vi "Protection_2.vi"() -> ()   [LabVIEW 2016]
uses:
  <vilib>/rvi/interface/nirviOpenFPGA/nirviOpenFPGA.xnode
  <vilib>/rvi/interface/nirviReadWriteControl/nirviReadWriteControl.xnode
  <vilib>/addons/Electrical Power/Basic/NI_EP_Basic.lvlib
  <vilib>/addons/Electrical Power/Basic/Measurement/RMS (N Channels).vi
  <vilib>/rvi/interface/nirviCloseFPGA/nirviCloseFPGA.xnode
  <vilib>/addons/Electrical Power/Basic/Measurement/Fundamental Vector (N Channels).vi
  FPGA Bitfiles/IntelliRupter2_FPGATarget.lvbitx
  <vilib>/FPGAPlugInAG/cRIO-9039 (Sync)/niLvFpga_Open_cRIO-9039 (Sync).vi
  <vilib>/rvi/interface/common/dynamic/niFpgaDynamicAddResources.vi
  <vilib>/rvi/interface/Simulation/niFpgaSimulationCallBeginRW.vi
  <vilib>/rvi/errors/niLvFpgaAdjustHostInterfaceError.vi
  <vilib>/FPGAPlugInAG/Dynamic/niLvFpga_Close_Dynamic.vi
  <vilib>/addons/Electrical Power/Protection/Definite Time Delay/subVIs/fpga_Time Delay Cfg.ctl
  <vilib>/addons/Electrical Power/Protection/NI_EP_Protection_FPGA.lvlib
panel:
  out "sum 2":dbl
  out "sum":dbl
  out "y":dbl[](array[numeric])
  out "x":dbl[](array[numeric])
  out "current fundamental vectors":cdb[](array[numeric])
  out "voltage fundamental vectors":cdb[](array[numeric])
  out "I array":waveform(sgl)[](array[waveform])=[{"t0"=timestamp(3615968248.53045 s since 1904-01-01), "dt"=1.736111111111111e-05, "Y"=array[1000 elements]}, {"t0"=timestamp(3615968248.53045 s since 1904-01-01), "dt"=1.736111111111111e-05, "Y"=array[1000 elements]}, {"t0"=timestamp(3615968248.53045 s since 1904-01-01), "dt"=1.736111111111111e-05, "Y"=array[1000 elements]}]
  out "VL array":waveform(sgl)[](array[waveform])=[{"t0"=timestamp(3615968248.53045 s since 1904-01-01), "dt"=1.736111111111111e-05, "Y"=array[1000 elements], "attributes"=variant("channel"=variant(enum16{"Va L", "Vb L", "Vc L", "Ia", "Ib", "Ic", "Va R", "Vb R", "Vc R"} enum."Va L"))}, {"t0"=timestamp(3615968248.53045 s since 1904-01-01), "dt"=1.736111111111111e-05, "Y"=array[1000 elements], "attributes"=variant("channel"=variant(enum16{"Va L", "Vb L", "Vc L", "Ia", "Ib", "Ic", "Va R", "Vb R", "Vc R"} enum."Vb L"))}, {"t0"=timestamp(3615968248.53045 s since 1904-01-01), "dt"=1.736111111111111e-05, "Y"=array[1000 elements], "attributes"=variant("channel"=variant(enum16{"Va L", "Vb L", "Vc L", "Ia", "Ib", "Ic", "Va R", "Vb R", "Vc R"} enum."Vc L"))}]
  in  "RMS minimum\nvalues":T1={"VRMS values"=[0.5, 0.5, 0.5], "IRMS values"=[0.1, 0.09999999999999998, 0.09999999999999998]}
  in  "Manual trip":bool
  in  "Relay7":bool
  in  "Reclose?":bool
  in  "Recloser Settings":T2={"Magnitude Minimum"=0.1, "Magnitude difference level"=0.1, "Frequency difference level"=0.1, "Phase difference level"=5.0}
  in  "time delay settings":T3={"operate time [ms]"=10, "reset time [ms]"=10, "operate time compensation [ms]"=10}
  out "VR error":i32
  out "VL error":i32
  in  "UV Reset level":dbl
  in  "Undervoltage \npick-up level":dbl=-1.0
  in  "OC Reset level":dbl=2.0
  in  "Overcurrent\npick-up level":dbl=100.0
  out "I error":i32
  in  "stop":bool
  out "half cycle (samples)":i32=96
  out "basic calc interval":u16=57600
  # "Overcurrent reset level should\nbe lower than pick-up level\n\nUndervoltage reset level should \nbe higher than pick-up level"
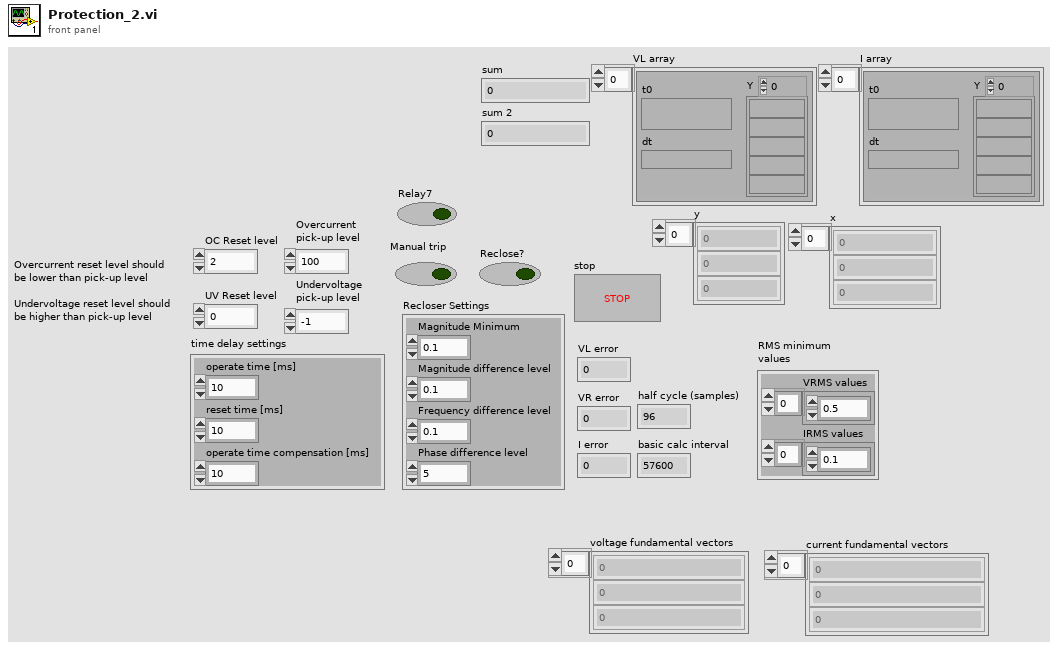
[diagram p1: front panel]
types:
  T1 = cluster{"VRMS values":dbl[], "IRMS values":dbl[]}
  T2 = cluster{"Magnitude Minimum":dbl, "Magnitude difference level":dbl, "Frequency difference level":dbl, "Phase difference level":dbl}
  T3 = typedef "NI_EP_Protection_FPGA.lvlib/fpga_Time Delay Cfg.ctl" = cluster{"operate time [ms]":u32, "reset time [ms]":u32, "operate time compensation [ms]":u32}
  T4 = typedef "NI_EP_Protection_FPGA.lvlib/fpga_Timer Feedback Var.ctl" = cluster{"time elapsed":u32, "start time of trip counting":u32, "start time of reseting":u32}
  T5 = typedef "NI_EP_Protection_FPGA.lvlib/fpga_State.ctl" = enum16{"Idle", "Trip Counting", "Tripped", "Reset Counting"}
  T6 = cluster{"timing values out":T4, "status out":T5, "trip signal out":bool}
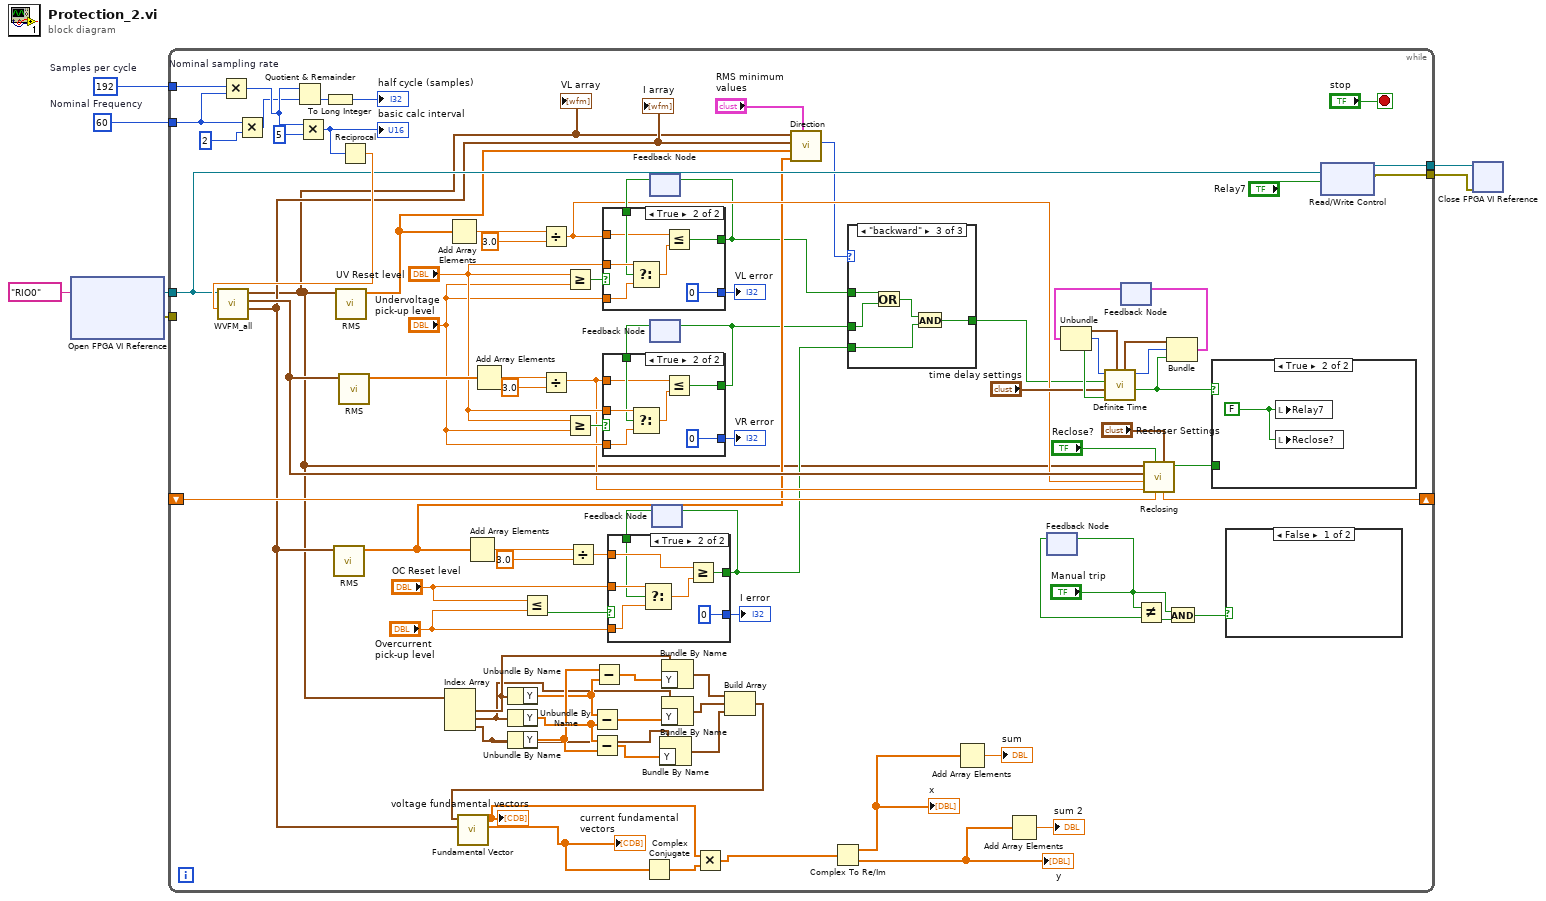
[diagram p0: block diagram]
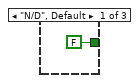
[diagram p2: hidden frame]
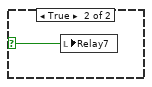
[diagram p5: hidden frame]
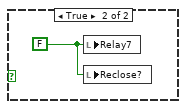
[diagram p6: hidden frame]
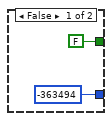
[diagram p7: hidden frame]
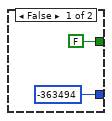
[diagram p8: hidden frame]
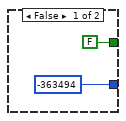
[diagram p9: hidden frame]
diagram:
  w3 = 192  # Samples per cycle
  w4 = 60  # Nominal Frequency
  n1 = xnode "Open FPGA VI Reference"("resource name"=tag "RIO0") -> ("FPGA VI Reference Out"=w7:refnum<k20>, "error out"=w6:errorcluster)  [unwired: 1 in]
  n2 = while {
    tunnel: w7 -> [w57]
    tunnel: w6 -> [_]
    tunnel: w4 -> [w88]
    tunnel: w3 -> [w87]
    shift-right: [w51] -> _
    shift-left: _ -> [w50]
    tunnel: [w49] -> w2
    tunnel: [w48] -> w1
    stop <- "stop" stop-if-true
    n3 = Multiply "Nominal sampling rate"(x=w87, y=w88) -> (x*y=w94:i32)
    n4 = Multiply(x=w88, y=2) -> (x*y=w90:i32)
    n5 = Quotient & Remainder(x=w94, y=w90) -> (floor(x/y)=w92:i32)  [unwired: 1 out]
    n6 = Multiply(x=w94, y=u16 5) -> (x*y=w95:i32)
    "basic calc interval" <- w95
    n7 = To Long Integer(number=w92) -> (32bit integer=→"half cycle (samples)":i32)
    n8 = Reciprocal(x=w95) -> (1/x=w85:dbl)
    n9 = call "WVFM_all.vi"("dt"=w85, "FPGA VI Reference"=w57) -> ("I array"=w30:waveform(sgl)[], "VR array"=w56:waveform(sgl)[], "VL array"=w15:waveform(sgl)[])  [unwired: 6 in]
    "VL array" <- w15
    "I array" <- w30
    n10 = call-poly <vilib>:"RMS.vi"("waveforms"=w30) -> ("RMS values"=w38:dbl[])  [unwired: 9 in, 1 out]
    n11 = call-poly <vilib>:"RMS.vi"("waveforms"=w15) -> ("RMS values"=w39:dbl[])  [unwired: 9 in, 1 out]
    n12 = call-poly <vilib>:"RMS.vi"("waveforms"=w56) -> ("RMS values"=w68:dbl[])  [unwired: 9 in, 1 out]
    n13 = Index Array(array=w15) -> (element #1=w23:waveform(sgl), element #2=w22:waveform(sgl), element #3=w20:waveform(sgl))  [unwired: 3 in]
    n14 = Add Array Elements(numeric array=w39) -> (sum=w76:dbl)
    n15 = Add Array Elements(numeric array=w38) -> (sum=w82:dbl)
    n16 = Add Array Elements(numeric array=w68) -> (sum=w71:dbl)
    n17 = Unbundle By Name(w23) -> ("Y"=w25:sgl[])
    n18 = Unbundle By Name(w22) -> ("Y"=w27:sgl[])
    n19 = Unbundle By Name(w20) -> ("Y"=w26:sgl[])
    n20 = Less Or Equal?(x="OC Reset level", y="Overcurrent\npick-up level") -> (x <= y?=w84:bool)
    n21 = Divide(x=w76, y=3.0) -> (x/y=w55:dbl)
    n22 = Divide(x=w71, y=3.0) -> (x/y=w54:dbl)
    n23 = Greater Or Equal?(x="UV Reset level", y="Undervoltage \npick-up level") -> (x >= y?=w79:bool)
    n24 = Greater Or Equal?(x="UV Reset level", y="Undervoltage \npick-up level") -> (x >= y?=w69:bool)
    n25 = Divide(x=w82, y=3.0 ("x")) -> (x/y=w81:dbl)
    n26 = Subtract(x=w25, y=w27) -> (x-y=w21:sgl[])
    n27 = Subtract(x=w27, y=w26) -> (x-y=w19:sgl[])
    n28 = Subtract(x=w26, y=w25) -> (x-y=w24:sgl[])
    n29 = feedback #1() -> (w77:bool)  [unwired: 1 in]
    n30 = case shown="True" w79 {
      tunnel: [FALSE w123] -> w35
      tunnel: [-363494 ("error") 0 ("error")] -> w74
      tunnel: "UV Reset level" -> [_ w121]
      tunnel: "Undervoltage \npick-up level" -> [_ w120]
      tunnel: w77 -> [_ w119]
      tunnel: w55 -> [_ w118]
      frame False {
      }
      frame True {
        n31 = Select(t=w121, s=w119, f=w120) -> (s? t:f=w124:dbl)
        n32 = Less Or Equal?(x=w118, y=w124) -> (x <= y?=w123:bool)
      }
    }
    "VL error" <- w74
    n33 = feedback-in #1(w35) -> ()
    n34 = feedback #2() -> (w70:bool)  [unwired: 1 in]
    n35 = case shown="True" w69 {
      tunnel: [FALSE w114] -> w34
      tunnel: [-363494 ("error") 0 ("error")] -> w73
      tunnel: "UV Reset level" -> [_ w112]
      tunnel: "Undervoltage \npick-up level" -> [_ w111]
      tunnel: w70 -> [_ w110]
      tunnel: w54 -> [_ w109]
      frame False {
      }
      frame True {
        n36 = Select(t=w112, s=w110, f=w111) -> (s? t:f=w115:dbl)
        n37 = Less Or Equal?(x=w109, y=w115) -> (x <= y?=w114:bool)
      }
    }
    "VR error" <- w73
    n38 = feedback-in #2(w34) -> ()
    n39 = feedback #3() -> (w78:bool)  [unwired: 1 in]
    n40 = case shown="True" w84 {
      tunnel: w81 -> [_ w133]
      tunnel: [-363494 ("error") 0 ("error")] -> w83
      tunnel: "OC Reset level" -> [_ w130]
      tunnel: "Overcurrent\npick-up level" -> [_ w129]
      tunnel: [FALSE ("Boolean") w128] -> w33
      tunnel: w78 -> [_ w127]
      frame False {
      }
      frame True {
        n41 = Select(t=w130, s=w127, f=w129) -> (s? t:f=w132:dbl)
        n42 = Greater Or Equal?(x=w133, y=w132) -> (x >= y?=w128:bool)
      }
    }
    "I error" <- w83
    n43 = feedback-in #3(w33) -> ()
    n44 = Bundle By Name(cluster=w20, "Y"=w19) -> (w17:waveform(sgl))
    n45 = Bundle By Name(cluster=w23, "Y"=w24) -> (w16:waveform(sgl))
    n46 = Bundle By Name(cluster=w22, "Y"=w21) -> (w18:waveform(sgl))
    n47 = Build Array(w16, w18, w17) -> (w14:waveform(sgl)[])
    n48 = call-poly <vilib>:"Fundamental Vector.vi"("current waveforms"=w30, "voltage waveforms"=w14) -> ("current fundamental vectors"=w12:cdb[], "voltage fundamental vectors"=w29:cdb[])  [unwired: 6 in, 2 out]
    "voltage fundamental vectors" <- w29
    "current fundamental vectors" <- w12
    n49 = Complex Conjugate(1:w12) -> (0:w13:cdb[])
    n50 = Multiply(x=w29, y=w13) -> (x*y=w28:cdb[])
    n51 = call "Direction.vi"("RMS minimum\nvalues"="RMS minimum\nvalues", "IRMS values"=w38, "VRMS values"=w39, "I array"=w30, "VL array"=w15) -> ("Direction"=w36:enum16{"forward", "backward", "N/D"})  [unwired: 6 in]
    n52 = Complex To Re/Im(x + iy=w28) -> (x=w11:dbl[], y=w10:dbl[])
    "x" <- w11
    "y" <- w10
    n53 = case shown="\"backward\"" w36 {
      tunnel: w35 -> [_ _ w102]
      tunnel: w34 -> [_ _ w101]
      tunnel: w33 -> [_ w97 w99]
      tunnel: [FALSE ("Boolean") w97 w98] -> w32
      frame "N/D", Default {
      }
      frame "forward" {
      }
      frame "backward" {
        n54 = Or(x=w102, y=w101) -> (x .or. y?=w100:bool)
        n55 = And(x=w100, y=w99) -> (x .and. y?=w98:bool)
      }
    }
    n56 = Add Array Elements(numeric array=w11) -> (sum=→"sum":dbl)
    n57 = Add Array Elements(numeric array=w10) -> (sum=→"sum 2":dbl)
    n58 = feedback #4() -> (w45:bool)  [unwired: 1 in]
    n59 = feedback-in #4("Manual trip") -> ()
    n60 = feedback #5() -> (w62:T6)  [unwired: 1 in]
    n61 = Unbundle(w62) -> ("timing values out"=w61:T4, "status out"=w60:T5, "trip signal out"=w59:bool)
    n62 = call "Definite Time.vi"("timing values in"=w61, "trip signal in"=w59, "time delay settings"="time delay settings", "pick-up signal? (F)"=w32, "status in"=w60) -> ("trip signal out"=w41:bool, "status out"=w64:T5, "timing values out"=w65:T4)  [unwired: 4 in]
    n63 = Not Equal?(x="Manual trip", y=w45) -> (x != y?=w44:bool)
    n64 = call "Reclosing.vi"("Recloser Settings"="Recloser Settings", "Counter In"=w50, "Reclose?"="Reclose?", "VR RMS avg"=w54, "VL RMS avg"=w55, "VR array"=w56, "VL array"=w15) -> ("Recloser action"=w40:bool, "Counter Out"=w51:dbl)  [unwired: 3 out]
    n65 = Bundle("timing values out"=w65, "status out"=w64, "trip signal out"=w41) -> (w63:T6)  [unwired: 1 in]
    n66 = feedback-in #5(w63) -> ()
    n67 = And(x="Manual trip", y=w44) -> (x .and. y?=w42:bool)
    n68 = case shown="True" w41 {
      tunnel: w40 -> [w103 _]
      frame False {
        n69 = case shown="False" w103 {
          selector: w103 -> [_ w104]
          frame False {
          }
          frame True {
            n70 = local write "Relay7"(w104) -> ()
          }
        }
      }
      frame True {
        w105 = FALSE ("Relay7")
        n71 = local write "Relay7"(w105) -> ()
        n72 = local write "Reclose?"(w105) -> ()
      }
    }
    n73 = case shown="False" w42 {
      frame False {
      }
      frame True {
        w106 = FALSE ("Relay7")
        n74 = local write "Relay7"(w106) -> ()
        n75 = local write "Reclose?"(w106) -> ()
      }
    }
    n76 = xnode "Read/Write Control"("FPGA VI Reference In"=w57, "Relay8"="Relay7") -> ("FPGA VI Reference Out"=w49:refnum<k20>, "error out"=w48:errorcluster)  [unwired: 1 in]
  }
  n77 = xnode "Close FPGA VI Reference"("FPGA VI Reference In"=w2, "error in"=w1) -> ()  [unwired: 1 out]
